vi "LiftMainSP.vi"(4 "Power":dbl, 8 "Error In":errorcluster, 9 "Reverse":bool, 10 "Forward":bool, 11 "Control Mode":enum16{"Open", "Control"}(ring)) -> (0 "Error Out":errorcluster)   [LabVIEW 2016]
uses:
  <vilib>/Rock Robotics/SystemInterfaces/DIO/FPGA_DIOPWMChannel.ctl
  <vilib>/Rock Robotics/WPI/MotorControl/WPI_MotorControlOpen VictorSP.vi
panel:
  # "Lift Control Main VI\nFRC Team 34"
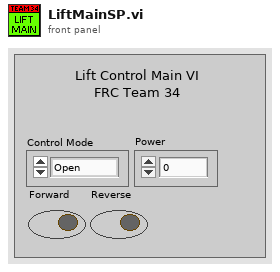
[diagram p1: front panel]
types:
  T1 = typedef "FPGA_DIOPWMChannel.ctl" = enum8{"PWM 0", "PWM 1", "PWM 2", "PWM 3", "PWM 4", "PWM 5", "PWM 6", "PWM 7", "PWM 8", "PWM 9", "PWM MXP 0", "PWM MXP 1", "PWM MXP 2", "PWM MXP 3", "PWM MXP 4", "PWM MXP 5", "PWM MXP 6", "PWM MXP 7", "PWM MXP 8", "PWM MXP 9", "Invalid"}
  T2 = typedef "WPI_MotorControlDeviceRef.ctl" = cluster{"DeviceStatus":errorcluster, "Type":T3, "PWM":cluster{"PWM Channel":T1, "DeadBand":T4}, "CAN":cluster{"Device Number":u8, "SetOutput VI Ref":variant, "GetOutput VI Ref":variant, "Enable VI Ref":variant, "Disable VI Ref":variant, "Data":variant}, "Invert":bool}
  T3 = typedef "WPI_MotorControlType.ctl" = enum16{"PWM", "CAN"}
  T4 = typedef "WPI_PWMDeadband.ctl" = cluster{"Name":string, "maxPositivePwm":i32, "minPositivePwm":i32, "centerPwm":i32, "maxNegativePwm":i32, "minNegativePwm":i32, "angularRange":u16}
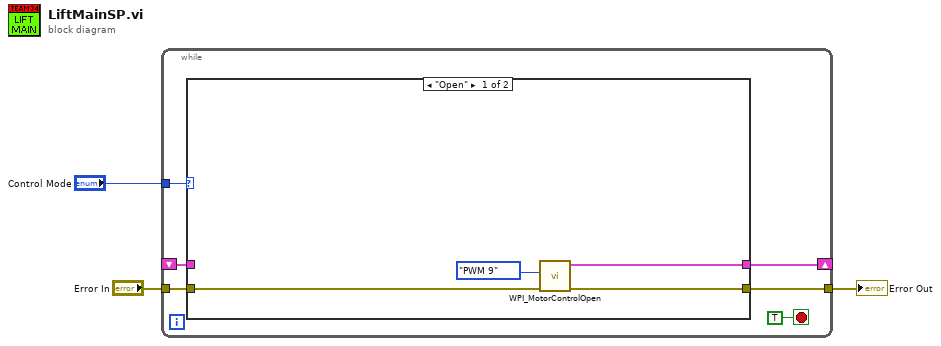
[diagram p0: block diagram]
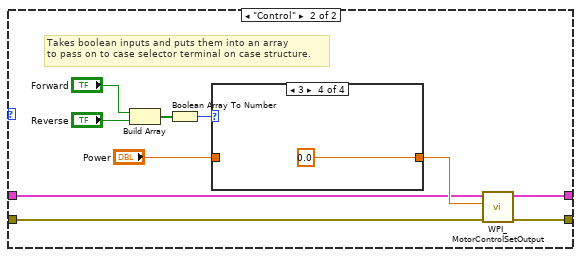
[diagram p2: hidden frame]
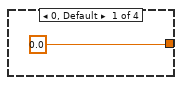
[diagram p3: hidden frame]
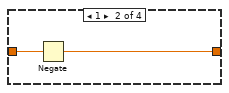
[diagram p4: hidden frame]
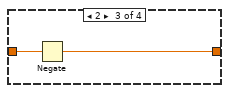
[diagram p5: hidden frame]
diagram:
  n1 = while {
    tunnel: "Control Mode" -> [w8]
    tunnel: "Error In" -> [w7]
    tunnel: [w6] -> w1
    shift-right: [w5] -> _
    shift-left: _ -> [w4]
    stop <- TRUE stop-if-true
    n2 = case shown="\"Open\"" w8 {
      tunnel: w7 -> [w13 w22]
      tunnel: [w10 w23] -> w6
      tunnel: [w11 w14] -> w5
      tunnel: w4 -> [_ w15]
      frame "Open" {
        n3 = call-poly <vilib>:"WPI_MotorControlOpen.vi"("error in (no error)"=w13, "PWM Channel"=FPGA_DIOPWMChannel."PWM 9") -> ("error out"=w10:errorcluster, "MotorControlDeviceRef"=w11:T2)  [unwired: 8 in]
      }
      frame "Control" {
        # "Takes boolean inputs and puts them into an array\nto pass on to case selector terminal on case structure."
        n4 = Build Array("Forward", "Reverse") -> (w18:bool[])
        n5 = Boolean Array To Number(Boolean array=w18) -> (number=w17:u32)
        n6 = case shown="3" w17 {
          tunnel: [0.0 ("RelayValue") w25 w27 0.0 ("RelayValue")] -> w16
          tunnel: "Power" -> [_ w26 w28 _]
          frame 0, Default {
          }
          frame 1 {
            n7 = Negate(x=w26) -> (-x=w25:dbl)
          }
          frame 2 {
            n8 = Negate(x=w28) -> (-x=w27:dbl)
          }
          frame 3 {
          }
        }
        n9 = call <vilib>:"WPI_MotorControlSetOutput.vi"("error in (no error)"=w22, "Output"=w16, "MotorControlDevRef"=w15) -> ("error out"=w23:errorcluster, "MotorControlDevRef"=w14:T2)  [unwired: 6 in, 1 out]
      }
    }
  }
  "Error Out" <- w1
